vi "Pockels-Control voltage.vi"(9 "Imaging Protocol":T1, 11 "Index of Z-plane":i32) -> (1 "Laser power (%)":u8, 3 "Pockels control voltage (V)":dbl)   [LabVIEW 2020]
uses:
  Typedefs/Imaging Protocols enum.ctl
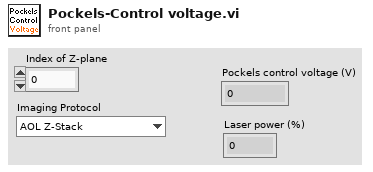
[diagram p1: front panel]
types:
  T1 = typedef "Imaging Protocols enum.ctl" = enum16{"AOL Z-Stack", "Motor Z Stack", "Functional Acquisition", "Single Plane Acquisition", "Volume Acquisition", "Live Imaging", "Live Plane Imaging", "Live Volume Imaging"}
  T2 = typedef "AOL_Globals.ctl" = cluster{"Imaging Protocol":T1, "Number of POI":u16, "Number of Miniscans":u16, "Number of Trials":u16, "Number of Cycles ":u64, "# Averaged Frames":u16, "Laser power (%)":u8, "Pockels (V)":dbl, "Acquisition Length (sec)":dbl, "Fill time (us)":dbl, "POI Dwell time (us)":dbl, "Miniscan Dwell time per pixel (us)":dbl, "PMT 1":dbl, "PMT 2":dbl, "Back Apperture (mA)":dbl, "Frame Size":T3, "Center Frequency":dbl, "Field of View (norm)":dbl, "DwellTime (us)":dbl, "Wavelength (nm)":dbl, "Zoom":dbl, "AOL Z":dbl, "AOL Mode":T4, "GridXY":dbl, "GridZ":dbl, "TriggerPeriod (sec)":dbl, "Number of Pixels in Miniscan":u16, "Experiment folder path":path, "X centre":dbl, "Y centre":dbl, "Angle (degrees)":dbl, "Plane Mode":T5, "Threshold":u16[], "Regenerate Chirps":bool, "Rectangle ROI length (pixels)":u16, "Rectangle ROI height (pixels)":u16, "AOD fill":u16, "StartupDelay":i32, "Samples Wait after Trigger":u16, "Slip Cycle":u32, "Add Cycle":bool, "Functional Mode":T6, "Z Start":dbl, "Z Stop":dbl, "# Planes":i32, "Total Pixels":i32, "Variable Miniscan Pixels":u16[], "Use Variable Length":bool, "Use Variable Resolution":bool, "Laser power (%) at Z Start":u8, "Laser power (%) at Z Stop":u8, "Ref Z Step":i8, "Ref Dwell Time (us)":dbl, "Field of View (um)":dbl}
  T3 = typedef "Frame Size.ctl" = u16
  T4 = typedef "AOL modes.ctl" = enum16{"Raster", "Structural", "Pointing", "Mini Scan", "Alignment"}
  T5 = typedef "Plane Mode.ctl" = u16
  T6 = typedef "Functional Mode.ctl" = enum16{"Point", "Line", "Patch", "Plane", "Volume"}
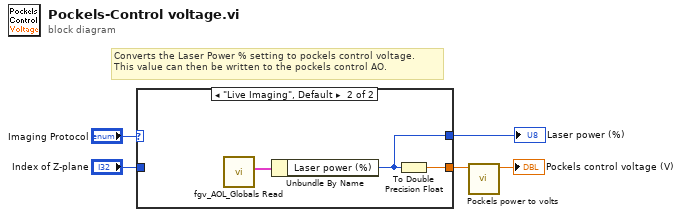
[diagram p0: block diagram]
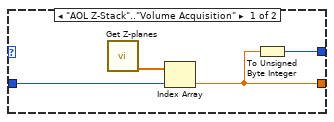
[diagram p2: hidden frame]
diagram:
  # "Converts the Laser Power % setting to pockels control voltage.\nThis value can then be written to the pockels control AO."
  n1 = case shown="\"Live Imaging\", Default" "Imaging Protocol" {
    tunnel: [w7 w11] -> w5
    tunnel: "Index of Z-plane" -> [w8 _]
    tunnel: [w6 w10] -> w1
    frame "AOL Z-Stack".."Volume Acquisition" {
      n2 = call "Get Z-planes.vi"() -> ("Pockels vs. Z (Laser power %)"=w9:dbl[])  [unwired: 7 in, 4 out]
      n3 = Index Array(array=w9, index=w8) -> (element=w7:dbl)
      n4 = To Unsigned Byte Integer(number=w7) -> (unsigned 8bit integer=w6:u8)
    }
    frame "Live Imaging", Default {
      n5 = call "fgv_AOL_Globals Read.vi"() -> ("AOL_Globals"=w12:T2)  [unwired: 9 in, 2 out]
      n6 = Unbundle By Name(w12) -> ("Laser power (%)"=w10:u8)
      n7 = To Double Precision Float(number=w10) -> (double precision float=w11:dbl)
    }
  }
  "Laser power (%)" <- w1
  n8 = call "Pockels power to volts.vi"("Pockels power (%)"=w5) -> ("Pockels control voltage (V)"=→"Pockels control voltage (V)":dbl)  [unwired: 8 in, 2 out]
